vi "rank plate.vi"(11 "plate arr":u8[][](array[numeric])) -> (3 "total point of plate":u32)   [LabVIEW 2024]
panel:
  in  "is there blocks":u32[][](array[numeric])
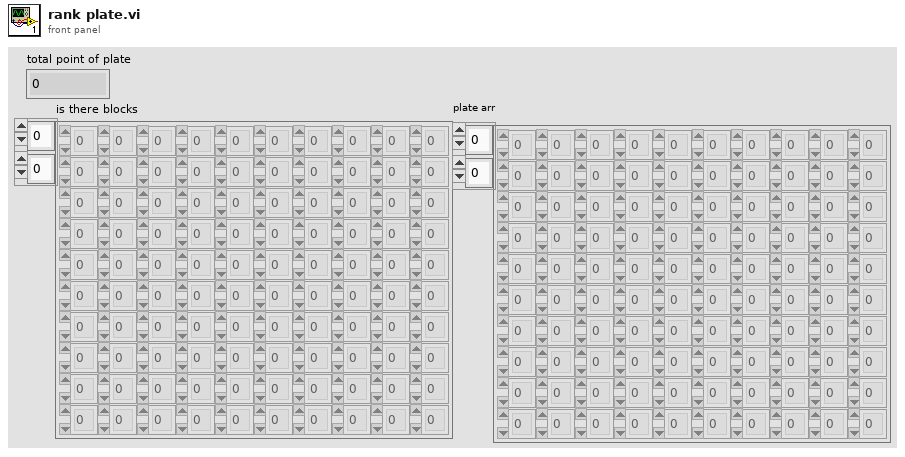
[diagram p1: front panel]
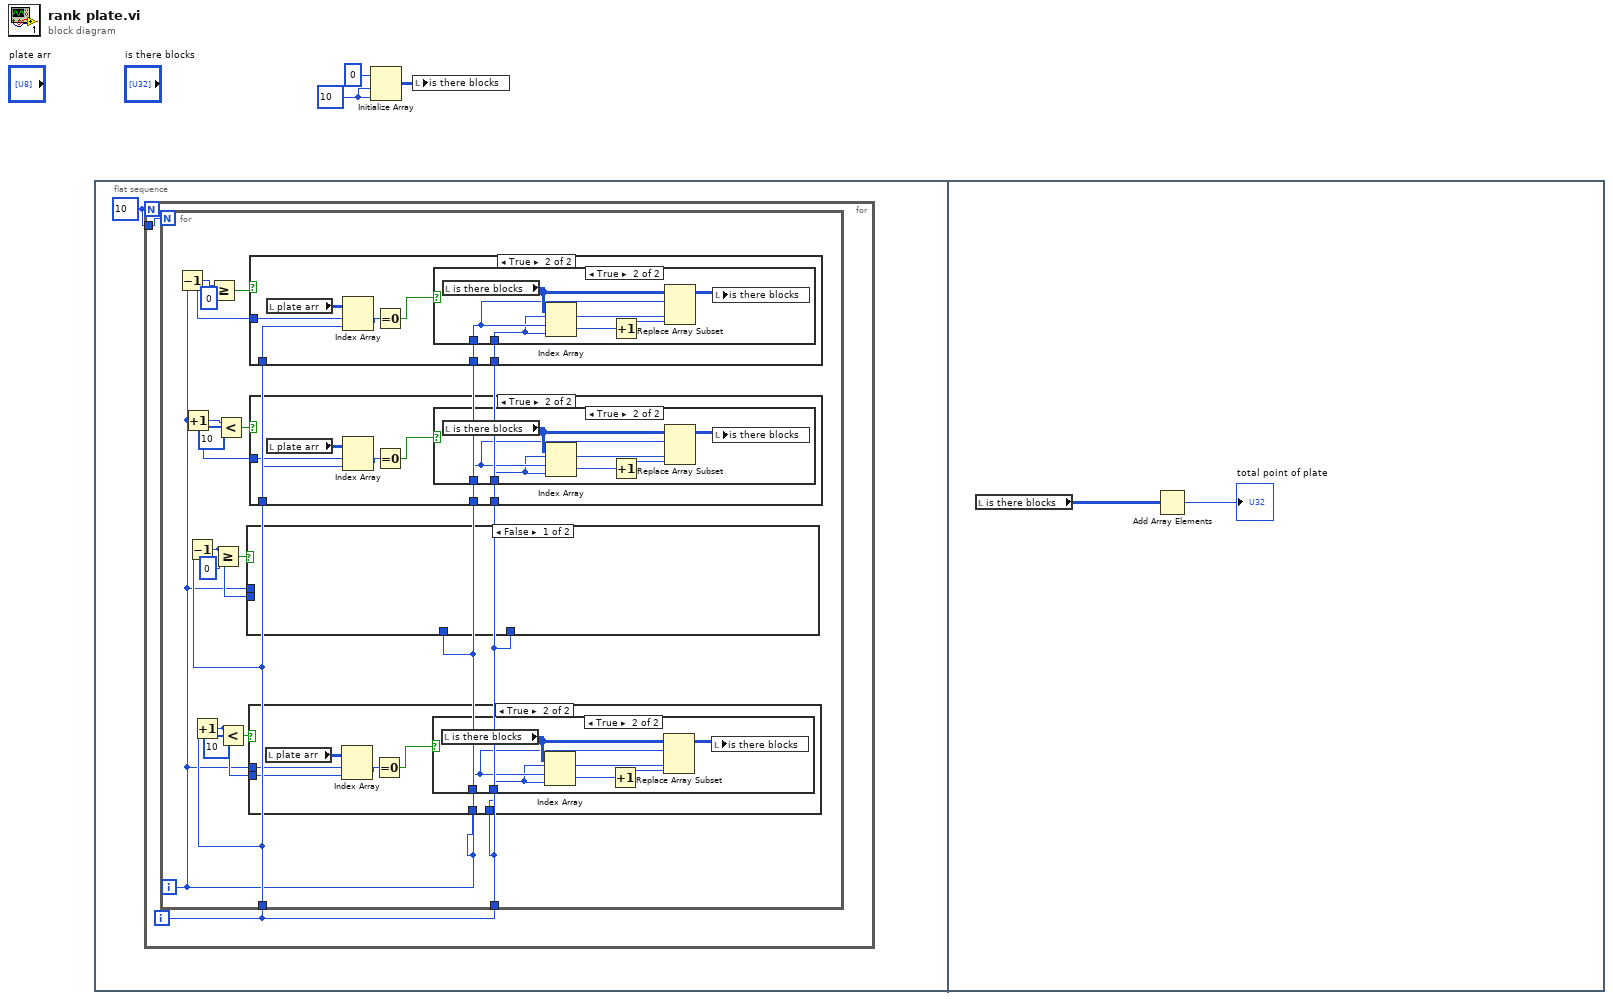
[diagram p0: block diagram]
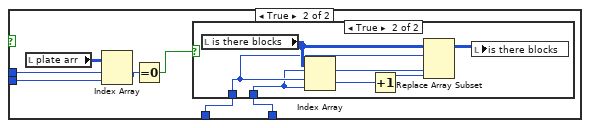
[diagram p4: hidden frame]
diagram:
  w3 = 10
  n1 = flat-sequence {
    frame #0 {
      w4 = 10
      n2 = for {
        N: w4 -> [_]
        tunnel: w4 -> [w5]
        i -> [w6]
        n3 = for {
          N: w5 -> [_]
          tunnel: w6 -> [w9]
          tunnel: w6 -> [w7]
          i -> [w8]
          n4 = Decrement(x=w8) -> (x-1=w19:i32)
          n5 = Increment(x=w8) -> (x+1=w17:i32)
          n6 = Decrement(x=w9) -> (x-1=w13:i32)
          n7 = Increment(x=w9) -> (x+1=w10:i32)
          n8 = Greater Or Equal?(x=w19, y=0) -> (x >= y?=w20:bool)
          n9 = Greater Or Equal?(x=w13, y=0) -> (x >= y?=w14:bool)
          n10 = Less?(x=w17, y=10) -> (x < y?=w16:bool)
          n11 = Less?(x=w10, y=10) -> (x < y?=w11:bool)
          n12 = case shown="False" w14 {
            tunnel: w13 -> [_ w38]
            tunnel: w8 -> [_ w37]
            tunnel: w7 -> [_ w36]
            tunnel: w8 -> [_ w35]
            frame False {
            }
            frame True {
              n13 = local read "plate arr"() -> (w39:u8[][])
              n14 = Index Array(array=w39, index (row)=w37, index (col)=w38) -> (element=w41:u8)
              n15 = Equal To 0?(x=w41) -> (x = 0?=w40:bool)
              n16 = case shown="True" w40 {
                tunnel: w35 -> [_ w44]
                tunnel: w36 -> [_ w43]
                frame False {
                }
                frame True {
                  n17 = local read "is there blocks"() -> (w45:u32[][])
                  n18 = Index Array(array=w45, index (row)=w44, index (col)=w43) -> (element=w47:u32)
                  n19 = Increment(x=w47) -> (x+1=w46:u32)
                  n20 = Replace Array Subset(array=w45, new element=w46, index (row)=w44, index (col)=w43) -> (w42:u32[][])
                  n21 = local write "is there blocks"(w42) -> ()
                }
              }
            }
          }
          n22 = case shown="True" w11 {
            tunnel: w10 -> [_ w25]
            tunnel: w8 -> [_ w24]
            tunnel: w8 -> [_ w23]
            tunnel: w7 -> [_ w22]
            frame False {
            }
            frame True {
              n23 = local read "plate arr"() -> (w26:u8[][])
              n24 = Index Array(array=w26, index (row)=w24, index (col)=w25) -> (element=w28:u8)
              n25 = Equal To 0?(x=w28) -> (x = 0?=w27:bool)
              n26 = case shown="True" w27 {
                tunnel: w23 -> [_ w31]
                tunnel: w22 -> [_ w30]
                frame False {
                }
                frame True {
                  n27 = local read "is there blocks"() -> (w32:u32[][])
                  n28 = Index Array(array=w32, index (row)=w31, index (col)=w30) -> (element=w34:u32)
                  n29 = Increment(x=w34) -> (x+1=w33:u32)
                  n30 = Replace Array Subset(array=w32, new element=w33, index (row)=w31, index (col)=w30) -> (w29:u32[][])
                  n31 = local write "is there blocks"(w29) -> ()
                }
              }
            }
          }
          n32 = case shown="True" w20 {
            tunnel: w19 -> [_ w67]
            tunnel: w9 -> [_ w66]
            tunnel: w8 -> [_ w62]
            tunnel: w7 -> [_ w61]
            frame False {
            }
            frame True {
              n33 = local read "plate arr"() -> (w63:u8[][])
              n34 = Index Array(array=w63, index (row)=w67, index (col)=w66) -> (element=w65:u8)
              n35 = Equal To 0?(x=w65) -> (x = 0?=w64:bool)
              n36 = case shown="True" w64 {
                tunnel: w62 -> [_ w70]
                tunnel: w61 -> [_ w69]
                frame False {
                }
                frame True {
                  n37 = local read "is there blocks"() -> (w71:u32[][])
                  n38 = Index Array(array=w71, index (row)=w70, index (col)=w69) -> (element=w73:u32)
                  n39 = Increment(x=w73) -> (x+1=w72:u32)
                  n40 = Replace Array Subset(array=w71, new element=w72, index (row)=w70, index (col)=w69) -> (w68:u32[][])
                  n41 = local write "is there blocks"(w68) -> ()
                }
              }
            }
          }
          n42 = case shown="True" w16 {
            tunnel: w17 -> [_ w54]
            tunnel: w9 -> [_ w53]
            tunnel: w8 -> [_ w49]
            tunnel: w7 -> [_ w48]
            frame False {
            }
            frame True {
              n43 = local read "plate arr"() -> (w50:u8[][])
              n44 = Index Array(array=w50, index (row)=w54, index (col)=w53) -> (element=w52:u8)
              n45 = Equal To 0?(x=w52) -> (x = 0?=w51:bool)
              n46 = case shown="True" w51 {
                tunnel: w49 -> [_ w57]
                tunnel: w48 -> [_ w56]
                frame False {
                }
                frame True {
                  n47 = local read "is there blocks"() -> (w58:u32[][])
                  n48 = Index Array(array=w58, index (row)=w57, index (col)=w56) -> (element=w60:u32)
                  n49 = Increment(x=w60) -> (x+1=w59:u32)
                  n50 = Replace Array Subset(array=w58, new element=w59, index (row)=w57, index (col)=w56) -> (w55:u32[][])
                  n51 = local write "is there blocks"(w55) -> ()
                }
              }
            }
          }
        }
      }
    }
    frame #1 {
      n52 = local read "is there blocks"() -> (w75:u32[][])
      n53 = Add Array Elements(numeric array=w75) -> (sum=→"total point of plate":u32)
    }
  }
  n54 = Initialize Array(0 ("element"), w3, w3) -> (w1:i32[][])
  n55 = local write "is there blocks"(w1) -> ()
